vi "Img_store.vi"(0 "total":i32, 1 "img_in":T1, 3 "img_data":dbl[][](array[numeric]), 4 "save":bool, 5 "Path":path) -> (2 "img_one":dbl[][](array[numeric]))   [LabVIEW 2016]
uses:
  <vilib>/vision/Image Controls.llb/IMAQ Image.ctl
panel:
  # "img out"
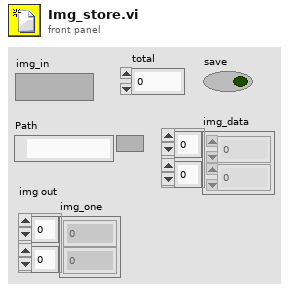
[diagram p1: front panel]
types:
  T1 = typedef "IMAQ Image.ctl" = refnum<image>
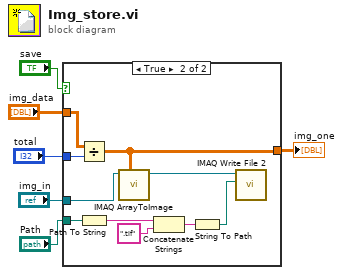
[diagram p0: block diagram]
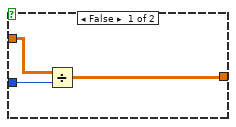
[diagram p2: hidden frame]
diagram:
  n1 = case shown="True" "save" {
    tunnel: "img_data" -> [w9 w19]
    tunnel: "Path" -> [_ w13]
    tunnel: "img_in" -> [_ w17]
    tunnel: "total" -> [w8 w16]
    tunnel: [w7 w10] -> w1
    frame False {
      n2 = Divide(x=w9, y=w8) -> (x/y=w7:dbl[][])
    }
    frame True {
      n3 = Divide(x=w19, y=w16) -> (x/y=w10:dbl[][])
      n4 = Path To String(path=w13) -> (string=w14:string)
      n5 = call "IMAQ ArrayToImage"("Image Pixels (U16)"=w10, "Image"=w17) -> ("Image Out"=w18:T1)  [unwired: 8 in, 1 out]
      n6 = Concatenate Strings(w14, ".tif" ("regular expression (\"\")")) -> (w15:string)
      n7 = String To Path(string=w15) -> (path=w12:path)
      n8 = call-poly "IMAQ Write File 2"("File Path"=w12, "Image"=w18) -> ()  [unwired: 8 in, 2 out]
    }
  }
  "img_one" <- w1
